vi "LVIS_Status.vi"(8 "Error In":errorcluster) -> (0 "Error Out":errorcluster)   [LabVIEW 2015]
doc: "Hidden process that monitors the SAF state, restores data from the backup file and displays messages to the user."
uses:
  Ctrls/LVIS_SAF Status.ctl
  Ctrls/LVIS_Msg State.ctl
  Globals/LVIS_DcGlobals.vi
panel:
  out "SAF State":T1=99 items=["Clear"=0, "SAF Active"=100, "SAF Complete"=101, "SAF > 50%"=102, "SAF < 50%"=103, "SAF Full"=104, "Unknown"=99]
  out "Last Update":timestamp
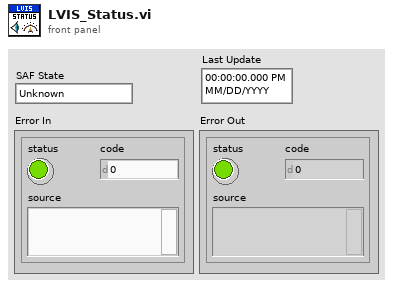
[diagram p1: front panel]
types:
  T1 = typedef "LVIS_SAF Status.ctl" = u16
  T2 = enum32{"Invalid", "Standard", "Closed", "Hidden", "Minimized", "Maximized"}
  T3 = typedef "LVIS_Msg State.ctl" = enum16{"None", "Offline", "Online", "Backup Full"}
  T4 = cluster{"PollRate":string, "ConnTimeout":string, "TxTimeout":string, "RxTimeout":string, "Port":string, "Map":string}
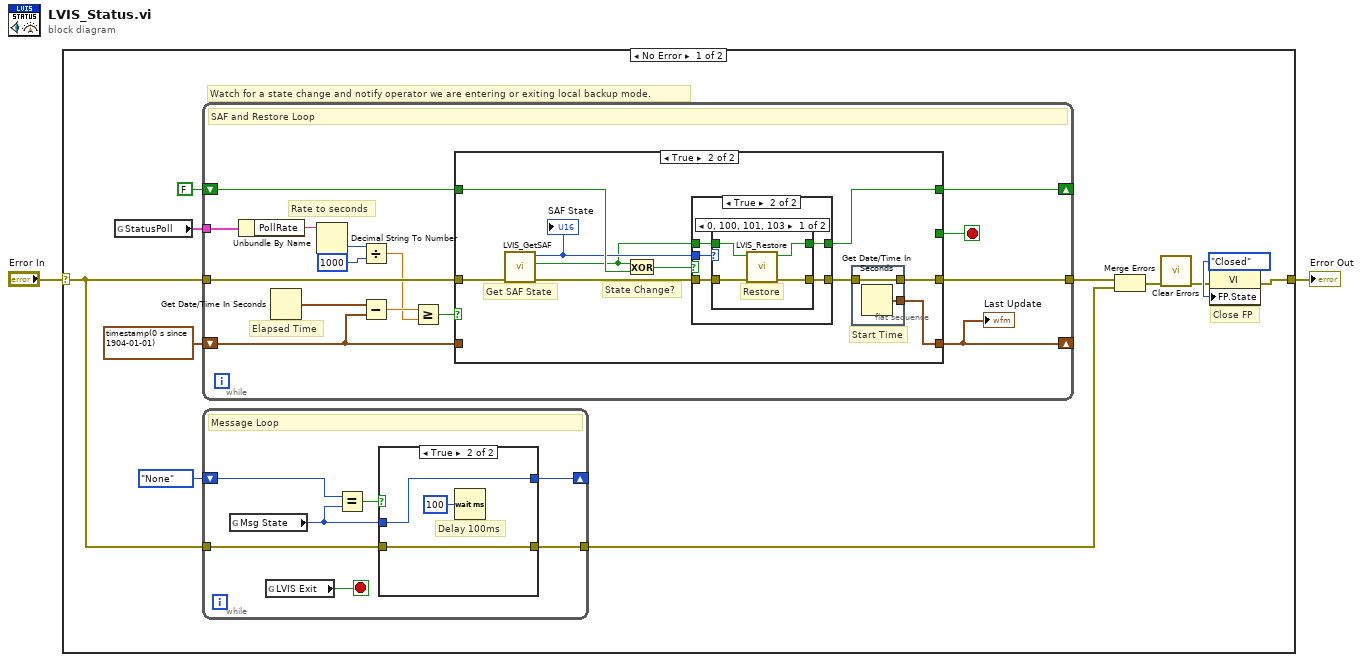
[diagram p0: block diagram]
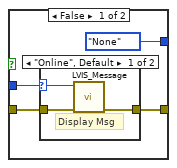
[diagram p2: hidden frame]
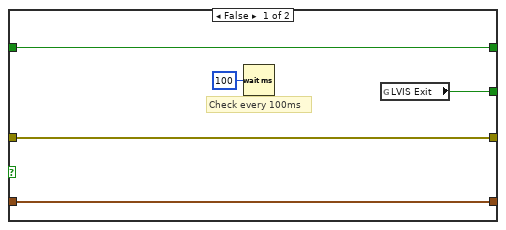
[diagram p4: hidden frame]
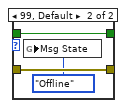
[diagram p6: hidden frame]
diagram:
  n1 = case shown="No Error" "Error In" {
    selector: "Error In" -> [w9 w78]
    tunnel: [w3 w78] -> w1
    frame No Error {
      # "Close FP"
      # "Watch for a state change and notify operator we are entering or exiting local backup mode."
      n2 = global read "LVIS_DcGlobals.vi" "StatusPoll"() -> (w10:T4)
      n3 = while {
        tunnel: w9 -> [w46]
        shift-right: [w45] -> _
        shift-left: FALSE ("Up?") -> [w44]
        tunnel: [w43] -> w12
        shift-right: [w33] -> _
        shift-left: timestamp(0 s since 1904-01-01) ("seconds since 1Jan1904") -> [w35]
        tunnel: w10 -> [w32]
        stop <- w34 stop-if-true
        # "Rate to seconds"
        # "Elapsed Time"
        # "SAF and Restore Loop"
        n4 = Unbundle By Name(w32) -> ("PollRate"=w41:string)
        n5 = Get Date/Time In Seconds() -> (seconds since 1Jan1904=w42:timestamp)
        n6 = Decimal String To Number(string=w41) -> (number=w40:i32)  [unwired: 2 in, 1 out]
        n7 = Divide(x=w40, y=1000) -> (x/y=w37:dbl)
        n8 = Subtract(x=w42, y=w35) -> (x-y=w38:dbl)
        n9 = Greater Or Equal?(x=w38, y=w37) -> (x >= y?=w36:bool)
        n10 = case shown="True" w36 {
          tunnel: w46 -> [w51 w61]
          tunnel: [w48 w52] -> w45
          tunnel: w44 -> [w48 w60]
          tunnel: [w51 w56] -> w43
          tunnel: [w50 w55] -> w33
          tunnel: w35 -> [w50 _]
          tunnel: [w49 _] -> w34
          frame False {
            # "Check every 100ms"
            n11 = Wait (ms)(milliseconds to wait=u32 100) -> ()  [unwired: 1 out]
            n12 = global read "LVIS_DcGlobals.vi" "LVIS Exit"() -> (w49:bool)
          }
          frame True {
            # "Start Time"
            # "State Change?"
            # "Get SAF State"
            n13 = call "LVIS_GetSAF.vi"("Error In"=w61) -> ("Error out"=w59:errorcluster, "Online?"=w53:bool, "SAF State"=w54:T1)  [unwired: 8 in]
            "SAF State" <- w54
            n14 = Exclusive Or(1:w60, 2:w53) -> (0:w58:bool)
            n15 = case shown="True" w58 {
              tunnel: w59 -> [w65 w70]
              tunnel: [w65 w69] -> w57
              tunnel: w54 -> [_ w68]
              tunnel: w53 -> [w64 w67]
              tunnel: [w64 w66] -> w52
              frame False {
                # "No Change in State"
              }
              frame True {
                n16 = case shown="0, 100, 101, 103" w68 {
                  tunnel: w70 -> [w74 w76]
                  tunnel: [w73 w76] -> w69
                  tunnel: w67 -> [w72 w77]
                  tunnel: [w71 w77] -> w66
                  frame 0, 100, 101, 103 {
                    # "Restore"
                    n17 = call "LVIS_Restore.vi"("Error In"=w74, "Online? In"=w72) -> ("Error Out"=w73:errorcluster, "Online? Out"=w71:bool)  [unwired: 8 in]
                  }
                  frame 99, Default {
                    n18 = global write "LVIS_DcGlobals.vi" "Msg State"(LVIS_Msg_State."Offline" ("Msg State")) -> ()
                  }
                }
              }
            }
            n19 = flat-sequence {
              tunnel: w57 -> [w63]
              tunnel: [w63] -> w56
              tunnel: [w62] -> w55
              frame #0 {
                n20 = Get Date/Time In Seconds() -> (seconds since 1Jan1904=w62:timestamp)
              }
            }
          }
        }
        "Last Update" <- w33
      }
      n21 = while {
        shift-right: [w17] -> _
        shift-left: LVIS_Msg_State."None" ("Msg State") -> [w18]
        tunnel: w9 -> [w20]
        tunnel: [w16] -> w8
        stop <- w14 stop-if-true
        # "Message Loop"
        n22 = global read "LVIS_DcGlobals.vi" "Msg State"() -> (w15:T3)
        n23 = global read "LVIS_DcGlobals.vi" "LVIS Exit"() -> (w14:bool)
        n24 = Equal?(x=w18, y=w15) -> (x = y?=w19:bool)
        n25 = case shown="True" w19 {
          tunnel: w20 -> [w24 w30]
          tunnel: [LVIS_Msg_State."None" ("Msg State") w29] -> w17
          tunnel: [w23 w30] -> w16
          tunnel: w15 -> [w21 w29]
          frame False {
            n26 = case shown="\"Online\", Default" w21 {
              selector: w21 -> [w25 _]
              tunnel: w24 -> [w27 w28]
              tunnel: [w26 w28] -> w23
              frame "Online", Default {
                # "Display Msg"
                n27 = call "LVIS_Message.vi"("Error In"=w27, "Msg State"=w25) -> ("Error Out"=w26:errorcluster)  [unwired: 9 in]
              }
              frame "None" {
              }
            }
          }
          frame True {
            # "Delay 100ms"
            n28 = Wait (ms)(milliseconds to wait=u32 100) -> ()  [unwired: 1 out]
          }
        }
      }
      n29 = Merge Errors(w12, w8) -> (w5:errorcluster)
      n30 = call <vilib>:"Clear Errors.vi"("error in (no error)"=w5) -> ("error out"=w4:errorcluster)  [unwired: 5 in, 1 out]
      n31 = property class="VI"(error in=w4, "FP.State"=T2."Closed" ("Front Panel Window:State")) -> (error out=w3:errorcluster)  [unwired: 1 in, 1 out]
    }
    frame Error {
    }
  }
  "Error Out" <- w1
